vi "Messwert im Toleranz-Bereich.vi"(7 "Rohwert":sgl, 8 "Toleranz Grundkalibrierung":sgl, 9 "Toleranz in % letzte KAL":sgl, 10 "Prüfgas-Konzentration":sgl, 11 "Messwert":sgl) -> (0 "im Bereich":bool)   [LabVIEW 2020, in "ABB-EL3000.lvlib" / "Allgemeine VI.lvlib"]
uses:
  Allgemeine VI.lvlib
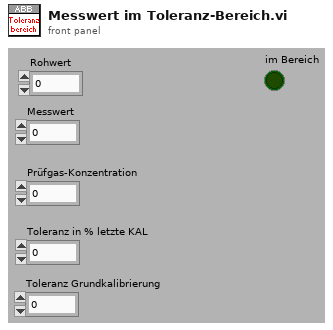
[diagram p1: front panel]
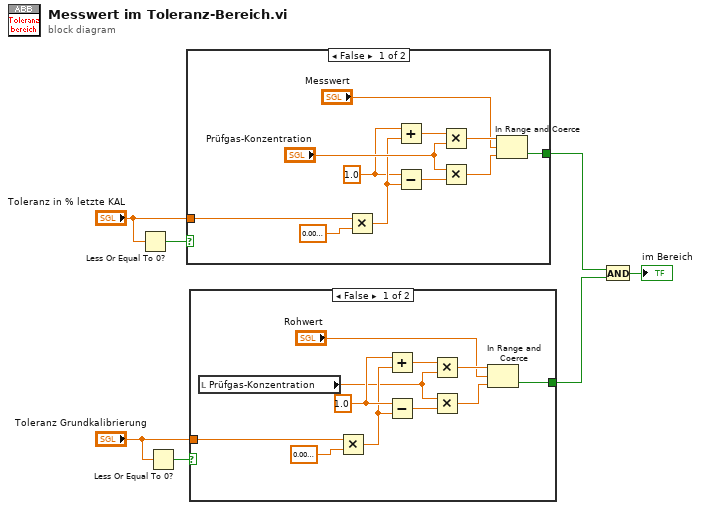
[diagram p0: block diagram]
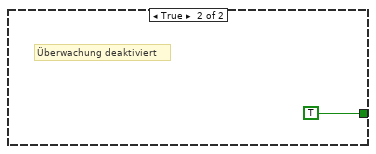
[diagram p2: hidden frame]
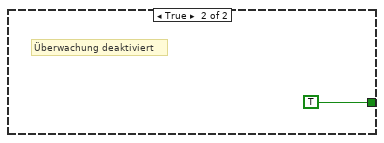
[diagram p3: hidden frame]
diagram:
  n1 = Less Or Equal To 0?(x="Toleranz in % letzte KAL") -> (x <= 0?=w1:bool)
  n2 = Less Or Equal To 0?(x="Toleranz Grundkalibrierung") -> (x <= 0?=w3:bool)
  n3 = case shown="False" w1 {
    tunnel: [w9 TRUE] -> w7
    tunnel: "Toleranz in % letzte KAL" -> [w8 _]
    frame False {
      w14 = sgl 1.0 ("x")
      n4 = Multiply(x=w8, y=sgl 0.01) -> (x*y=w15:sgl)
      n5 = Add(x=w14, y=w15) -> (x+y=w16:sgl)
      n6 = Subtract(x=w14, y=w15) -> (x-y=w17:sgl)
      n7 = Multiply(x=w16, y="Prüfgas-Konzentration") -> (x*y=w12:sgl)
      n8 = Multiply(x="Prüfgas-Konzentration", y=w17) -> (x*y=w13:sgl)
      n9 = In Range and Coerce(upper limit=w12, x="Messwert", lower limit=w13) -> (In Range?=w9:bool)  [unwired: 1 out]
    }
    frame True {
      # "Überwachung deaktiviert"
    }
  }
  n10 = case shown="False" w3 {
    tunnel: [w21 TRUE] -> w6
    tunnel: "Toleranz Grundkalibrierung" -> [w20 _]
    frame False {
      w27 = sgl 1.0 ("x")
      n11 = local read "Prüfgas-Konzentration"() -> (w22:sgl)
      n12 = Multiply(x=w20, y=sgl 0.01) -> (x*y=w26:sgl)
      n13 = Add(x=w27, y=w26) -> (x+y=w25:sgl)
      n14 = Subtract(x=w27, y=w26) -> (x-y=w24:sgl)
      n15 = Multiply(x=w25, y=w22) -> (x*y=w29:sgl)
      n16 = Multiply(x=w22, y=w24) -> (x*y=w28:sgl)
      n17 = In Range and Coerce(upper limit=w29, x="Rohwert", lower limit=w28) -> (In Range?=w21:bool)  [unwired: 1 out]
    }
    frame True {
      # "Überwachung deaktiviert"
    }
  }
  n18 = And(x=w7, y=w6) -> (x .and. y?=→"im Bereich":bool)
